vi "AM Configure Hardware.vi"(8 "error in (no error)":errorcluster, 11 "Hardware Resources in":T1) -> (0 "error out":errorcluster, 3 "Hardware Resources out":T1)   [LabVIEW 2020, in "Motion.lvlib"]
doc: "Configure the hardware."
uses:
  Motion.lvlib
  AM Configuration.ctl
  support/Message Queue/Message Cluster.ctl
  support/Message Queue/Message Queue.lvlib
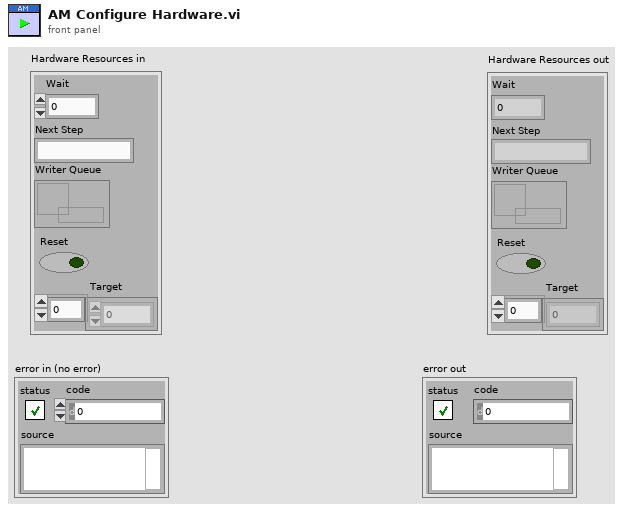
[diagram p1: front panel]
types:
  T1 = typedef "Motion.lvlib/AM Configuration.ctl" = cluster{"Wait":dbl, "Next Step":string, "Writer Queue":refnum<queue>, "Reset":bool, "Target":dbl[]}
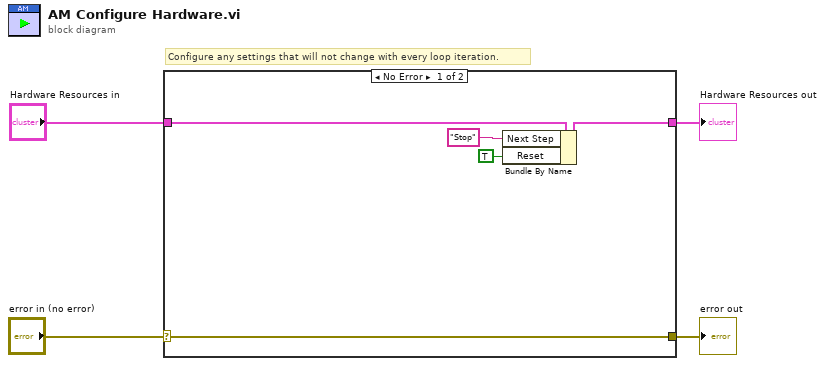
[diagram p0: block diagram]
diagram:
  # "Configure any settings that will not change with every loop iteration."
  n1 = case shown="No Error" "error in (no error)" {
    selector: "error in (no error)" -> [w9 w10]
    tunnel: [w9 w10] -> w3
    tunnel: "Hardware Resources in" -> [w6 w11]
    tunnel: [w8 w11] -> w1
    frame No Error {
      n2 = Bundle By Name(cluster=w6, "Next Step"="Stop", "Reset"=TRUE) -> (w8:T1)
    }
    frame Error {
    }
  }
  "Hardware Resources out" <- w1
  "error out" <- w3
